vi "write_return_std.vi"(8 "error in (no error)":errorcluster, 10 "return_std":bool, 11 "BayesianRidge in":refnum<class "BayesianRidge.lvclass">) -> (0 "error out":errorcluster, 3 "BayesianRidge out":refnum<class "BayesianRidge.lvclass">)   [LabVIEW 2020, in "BayesianRidge.lvclass"]
uses:
  BayesianRidge.lvclass
  BayesianRidge.lvclass/BayesianRidge.ctl
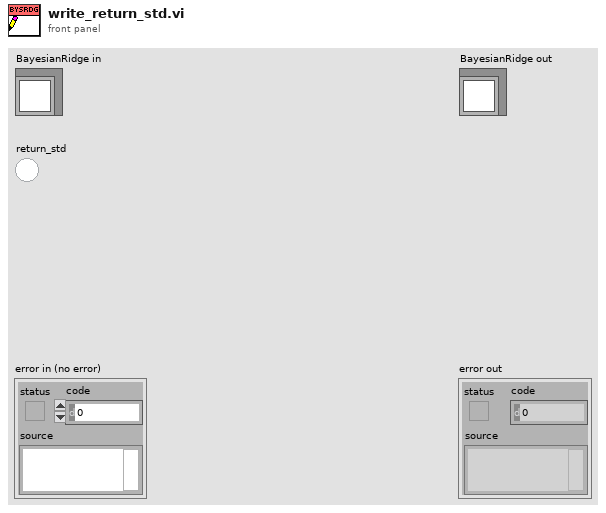
[diagram p1: front panel]
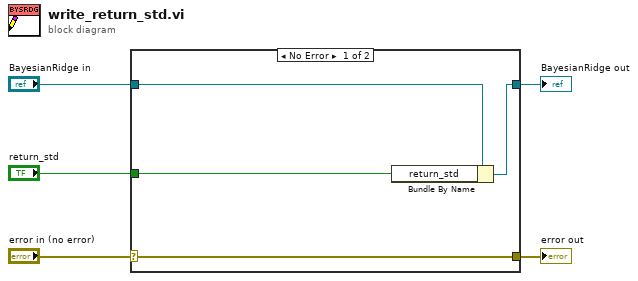
[diagram p0: block diagram]
diagram:
  n1 = case shown="No Error" "error in (no error)" {
    selector: "error in (no error)" -> [w9 w10]
    tunnel: [w9 w10] -> w4
    tunnel: [w7 w11] -> w2
    tunnel: "BayesianRidge in" -> [w8 w11]
    tunnel: "return_std" -> [w6 _]
    frame No Error {
      n2 = Bundle By Name(cluster=w8, "return_std"=w6) -> (w7:refnum<class "BayesianRidge.lvclass">)
    }
    frame Error {
    }
  }
  "error out" <- w4
  "BayesianRidge out" <- w2
